vi "UDP ROBO to CRIO.vi"() -> (0 "error out":errorcluster)   [LabVIEW 2016]
uses:
  Globale Variable/Globale Variable.vi
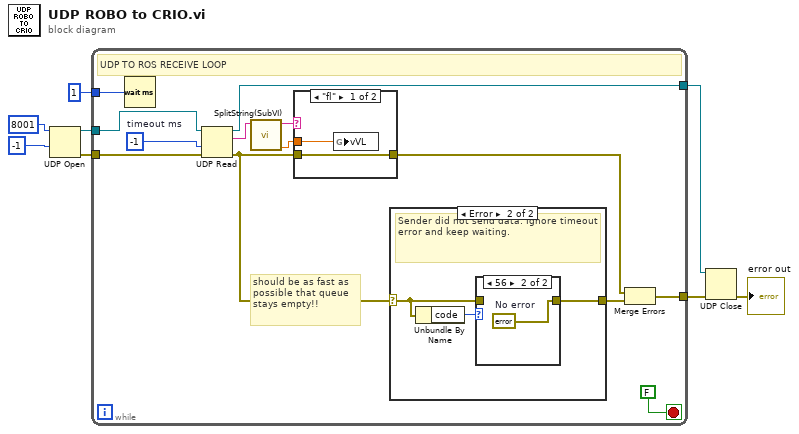
[diagram p0: block diagram]
diagram:
  n1 = UDP Open(9:-1 ("timeout ms (25000)"), 11:u16 8001 ("port")) -> (port=w5:refnum<k16>, 0:w8:errorcluster)  [unwired: 3 in, 1 out]
  n2 = while {
    tunnel: [w20] -> w2
    tunnel: u32 1 ("milliseconds to wait") -> [w16]
    tunnel: [w13] -> w4
    tunnel: w5 -> [w10]
    tunnel: w8 -> [w9]
    stop <- FALSE stop-if-true
    w21 = -1  # timeout ms
    # "should be as fast as possible that queue stays empty!!"
    # "UDP TO ROS RECEIVE LOOP"
    n3 = Wait (ms)(milliseconds to wait=w16) -> ()  [unwired: 1 out]
    n4 = UDP Read(connection ID=w10, timeout ms (25000)=w21, 8:w9) -> (data out=w17:string, error out=w12:errorcluster, 3:w20:refnum<k16>)  [unwired: 3 out]
    n5 = call "SplitString(SubVI).vi"("data in"=w17) -> ("Numeric"=w19:dbl, "String 3"=w18:string)  [unwired: 9 in]
    n6 = case shown="\"fl\"" w18 {
      tunnel: w19 -> [w22 _]
      tunnel: w12 -> [w23 w24]
      tunnel: [w23 w24] -> w14
      frame "fl" {
        n7 = global write "Globale Variable.vi" "vVL"(w22) -> ()
      }
      frame Default {
      }
    }
    n8 = case shown="Error" w12 {
      selector: w12 -> [w25 w27]
      tunnel: [w25 w26] -> w15
      frame No Error {
        # "Sender sent data. Update the chart value."
      }
      frame Error {
        # "Sender did not send data. Ignore timeout error and keep waiting."
        n9 = Unbundle By Name(w27) -> ("code"=w28:i32)
        n10 = case shown="56" w28 {
          tunnel: w27 -> [w29 _]
          tunnel: [w29 w30] -> w26
          frame Default {
          }
          frame 56 {
            w30 = errorcluster {"status"=FALSE, "code"=0, "source"=""}  # No error
          }
        }
      }
    }
    n11 = Merge Errors(w14, w15) -> (w13:errorcluster)
  }
  n12 = UDP Close(connection ID=w2, 8:w4) -> (error out=→"error out":errorcluster)  [unwired: 1 out]
